vi "add.vi"(0 "reference":refnum<class "Graph.lvclass">, 1 "node":refnum<class "AbstractNode.lvclass">, 2 "point":T1 {"y" format="%.2f"; "x" format="%.2f"}, 5 "error in (no error)":errorcluster) -> (14 "reference out":refnum<class "Graph.lvclass">, 15 "added":bool, 19 "error out":errorcluster)   [LabVIEW 2020, in "Graph.lvclass"]
doc: "public boolean add(Node n, Point2D p)"
uses:
  <resource>/Framework/Providers/Open_GDS/UML/Graph_class/Graph.lvclass
  <resource>/Framework/Providers/Open_GDS/UML/AbstractNode_class/AbstractNode.lvclass
  <resource>/Framework/Providers/Open_GDS/UML/General/Point/Point Point2D.ctl
  <resource>/Framework/Providers/Open_GDS/UML/RectangularNode_class/RectangularNode.lvclass
  C:/Program Files (x86)/National Instruments/LabVIEW 2020/resource/Framework/Providers/Open_GDS/UML/AbstractNode_class/AbstractNode.lvclass
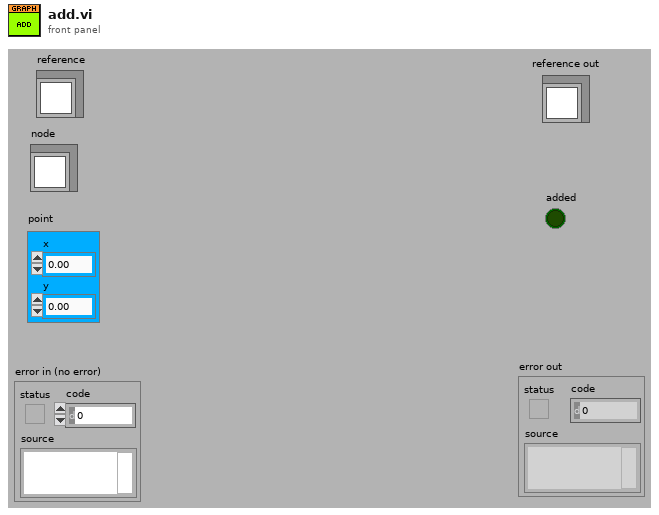
[diagram p1: front panel]
types:
  T1 = typedef "Point Point2D.ctl" = cluster{"x":dbl, "y":dbl}
  T2 = typedef "Graph.lvclass/ObjectAttributes.ctl" = cluster{"nodes":refnum<class "AbstractNode.lvclass">[], "edges":refnum<class "AbstractEdge.lvclass">[], "nodesToBeRemoved":refnum<class "AbstractNode.lvclass">[], "edgesToBeRemoved":refnum<class "AbstractEdge.lvclass">[], "needsLayout":bool, "LayoutNodes":refnum<class "AbstractNode.lvclass">[]}
  T3 = typedef "Rectangle Rectangle2D.ctl" = cluster{"x":dbl, "y":dbl, "width":dbl, "height":dbl}
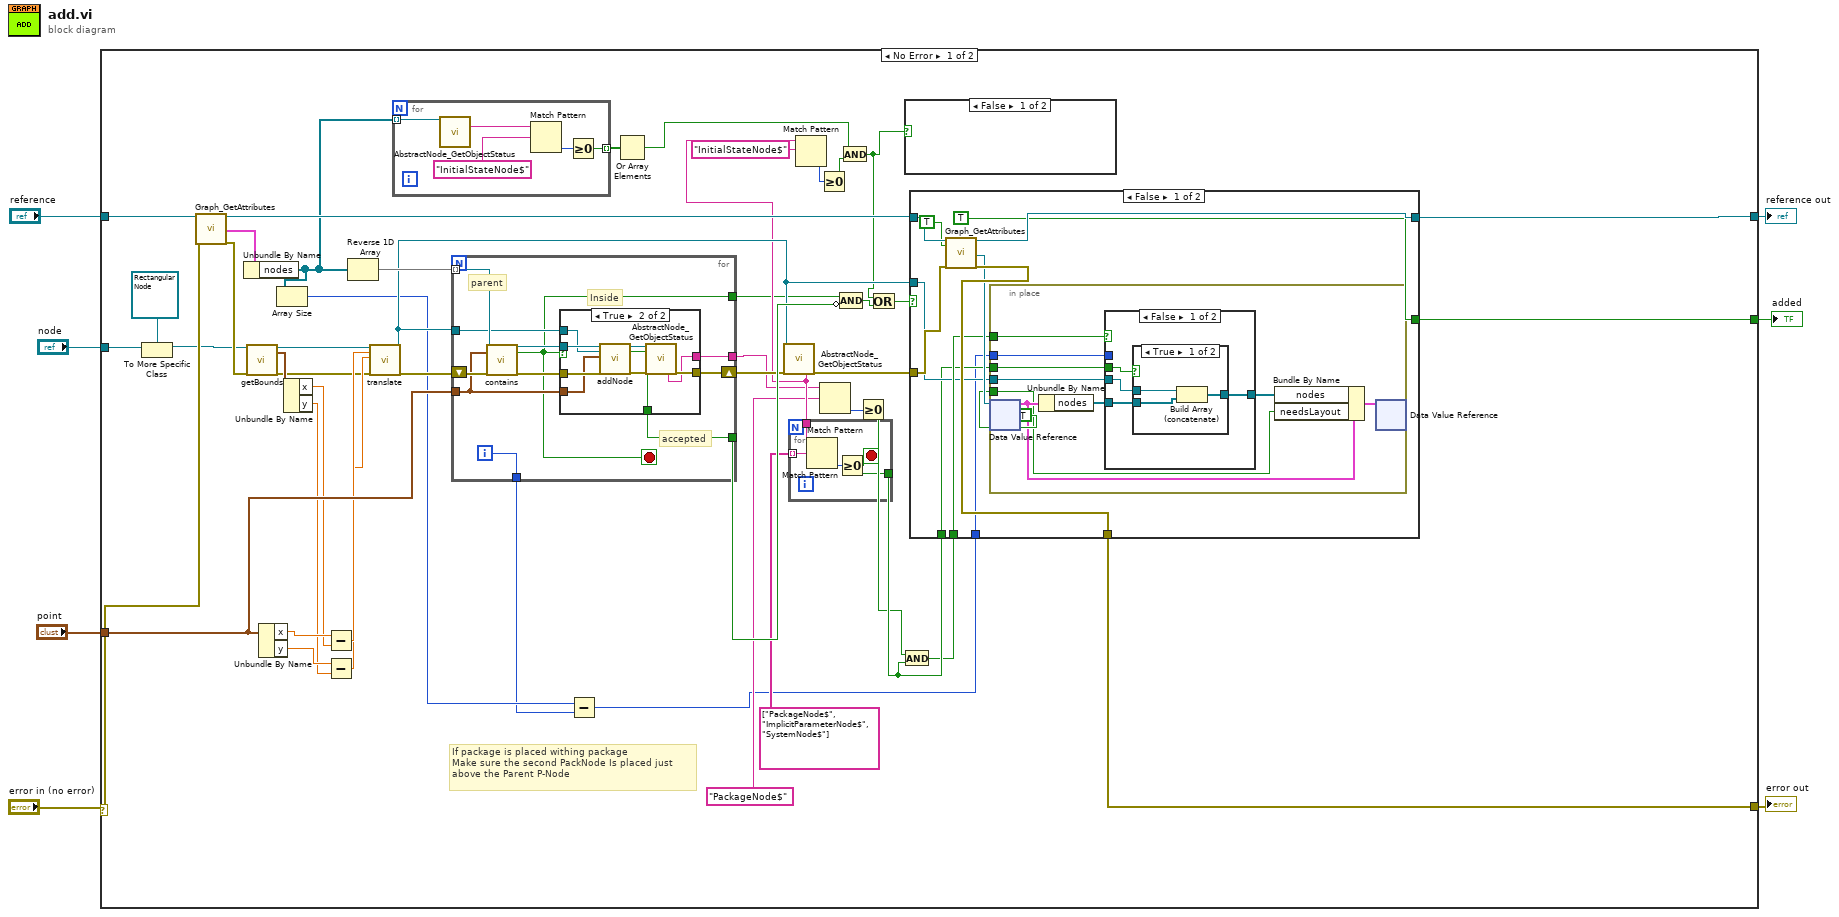
[diagram p0: block diagram]
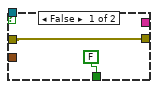
[diagram p2: hidden frame]
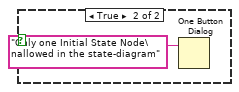
[diagram p3: hidden frame]
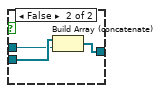
[diagram p4: hidden frame]
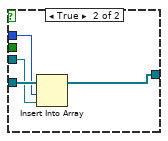
[diagram p5: hidden frame]
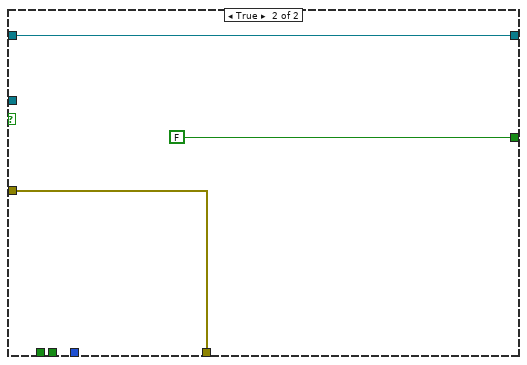
[diagram p6: hidden frame]
diagram:
  n1 = case shown="No Error" "error in (no error)" {
    selector: "error in (no error)" -> [w52 w126]
    tunnel: "reference" -> [w55 w127]
    tunnel: [w54 w126] -> w6
    tunnel: [w53 w127] -> w5
    tunnel: "node" -> [w21 _]
    tunnel: "point" -> [w51 _]
    tunnel: [w50 _] -> w1
    frame No Error {
      # "If package is placed withing package\nMake sure the second PackNode Is placed just\nabove the Parent P-Node"
      n2 = To More Specific Class(target class=refnum<class "RectangularNode.lvclass"> refnum ("reference"), reference=w21) -> (specific class reference=w19:refnum<class "RectangularNode.lvclass">)  [unwired: 1 in, 1 out]
      n3 = call <resource>:"Graph_GetAttributes.vi"("reference in"=w55, "error in (no error)"=w52) -> ("reference out"=w39:refnum<class "Graph.lvclass">, "Data"=w8:T2, "error out"=w36:errorcluster)  [unwired: 1 in, 14 out]
      n4 = Unbundle By Name(w8) -> ("nodes"=w30:refnum<class "AbstractNode.lvclass">[])
      n5 = call-dynamic "getBounds.vi"("reference"=w19, "error in (no error)"=w36) -> ("reference out"=w49:refnum<class "RectangularNode.lvclass">, "bounds"=w47:T3, "error out"=w41:errorcluster)  [unwired: 15 in]
      n6 = Unbundle By Name(w51) -> ("x"=w48:dbl, "y"=w44:dbl)
      n7 = Array Size(array=w30) -> (size(s)=w14:i32)
      n8 = Unbundle By Name(w47) -> ("x"=w46:dbl, "y"=w43:dbl)
      n9 = Subtract(x=w48, y=w46) -> (x-y=w45:dbl)
      n10 = Subtract(x=w44, y=w43) -> (x-y=w42:dbl)
      n11 = Reverse 1D Array(array=w30) -> (reversed array=w35:refnum<class "AbstractNode.lvclass">[])
      n12 = call-dynamic "translate.vi"("reference"=w49, "dx"=w45, "dy"=w42, "error in (no error)"=w41) -> ("reference out"=w32:refnum<class "RectangularNode.lvclass">, "error out"=w40:errorcluster)  [unwired: 14 in]
      n13 = for {
        tunnel: w30 -> [w83] mode=indexing
        tunnel: [w80] -> w27 mode=indexing
        n14 = call <resource>:"AbstractNode_GetObjectStatus.vi"("reference in"=w83) -> ("Class name"=w79:string)  [unwired: 1 in, 17 out]
        n15 = Match Pattern(string=w79, regular expression="InitialStateNode$" ("y")) -> (offset past match=w81:i32)  [unwired: 4 out]
        n16 = Greater Or Equal To 0?(x=w81) -> (x >= 0?=w80:bool)
      }
      n17 = for {
        shift-right: [w60] -> w34
        shift-left: w40 -> [w66]
        tunnel: w35 -> [w65] mode=indexing
        tunnel: [w56] -> w18
        tunnel: w32 -> [w62]
        tunnel: w51 -> [w61]
        tunnel: [w58] -> w38
        tunnel: [w59] -> w17
        tunnel: [w57] -> w13
        i -> [w57]
        stop <- w56 stop-if-true
        # "parent"
        # "accepted"
        # "Inside"
        n18 = call-dynamic "contains.vi"("reference"=w65, "point2D"=w61, "error in (no error)"=w66) -> ("reference out"=w63:refnum<class "AbstractNode.lvclass">, "contains"=w56:bool, "error out"=w64:errorcluster)  [unwired: 14 in]
        n19 = case shown="True" w56 {
          tunnel: w64 -> [w68 w77]
          tunnel: w63 -> [_ w76]
          tunnel: w62 -> [_ w75]
          tunnel: w61 -> [_ w74]
          tunnel: [w68 w71] -> w60
          tunnel: [FALSE ("added") w73] -> w58
          tunnel: [_ w69] -> w59
          frame False {
          }
          frame True {
            n20 = call-dynamic "addNode.vi"("reference"=w76, "node"=w75, "point2D"=w74, "error in (no error)"=w77) -> ("reference out"=w70:refnum<class "AbstractNode.lvclass">, "added"=w73:bool, "error out"=w72:errorcluster)  [unwired: 13 in]
            n21 = call <resource>:"AbstractNode_GetObjectStatus.vi"("reference in"=w70, "error in (no error)"=w72) -> ("Class name"=w69:string, "error out"=w71:errorcluster)  [unwired: 16 out]
          }
        }
      }
      n22 = Subtract(x=w14, y=w13) -> (x-y=w12:i32)
      n23 = Or Array Elements(Boolean array=w27) -> (logical OR=w24:bool)
      n24 = call <resource>:"AbstractNode_GetObjectStatus.vi"("reference in"=w32, "error in (no error)"=w34) -> ("Class name"=w29:string, "error out"=w33:errorcluster)  [unwired: 16 out]
      n25 = for {
        tunnel: [w84] -> w11
        tunnel: w29 -> [w86]
        tunnel: string[] ["PackageNode$", "ImplicitParameterNode$", "SystemNode$"] -> [w85] mode=indexing
        stop <- w84 stop-if-true
        n26 = Match Pattern(string=w86, regular expression=w85) -> (offset past match=w87:i32)  [unwired: 4 out]
        n27 = Greater Or Equal To 0?(x=w87) -> (x >= 0?=w84:bool)
      }
      n28 = Match Pattern(string=w29, regular expression="InitialStateNode$" ("y")) -> (offset past match=w26:i32)  [unwired: 4 out]
      n29 = Greater Or Equal To 0?(x=w26) -> (x >= 0?=w25:bool)
      n30 = Match Pattern(string=w17, regular expression="PackageNode$" ("y")) -> (offset past match=w15:i32)  [unwired: 4 out]
      n31 = And(x=w24, y=w25) -> (x .and. y?=w22:bool)
      n32 = Compound Arithmetic op=AND(w18, invert w38) -> (w37:bool)
      n33 = Greater Or Equal To 0?(x=w15) -> (x >= 0?=w10:bool)
      n34 = Or(x=w22, y=w37) -> (x .or. y?=w23:bool)
      n35 = And(x=w10, y=w11) -> (x .and. y?=w9:bool)
      n36 = case shown="False" w22 {
        frame False {
        }
        frame True {
          n37 = One Button Dialog(message="Only one Initial State Node\nallowed in the state-diagram") -> ()  [unwired: 2 out]
        }
      }
      n38 = case shown="False" w23 {
        tunnel: w39 -> [w99 w125]
        tunnel: [w98 w125] -> w53
        tunnel: [TRUE ("needsLayout") FALSE] -> w50
        tunnel: w33 -> [w95 w123]
        tunnel: [w96 w123] -> w54
        tunnel: w32 -> [w90 _]
        tunnel: w11 -> [w89 _]
        tunnel: w12 -> [w88 _]
        tunnel: w9 -> [w91 _]
        frame False {
          n39 = call <resource>:"Graph_GetAttributes.vi"("reference in"=w99, "OnlyGetDvrReference(False)"=TRUE, "error in (no error)"=w95) -> ("reference out"=w98:refnum<class "Graph.lvclass">, "DataRef"=w93:refnum<data-value>, "error out"=w96:errorcluster)  [unwired: 13 in, 1 out]
          n40 = in-place {
            in-place-border: TRUE ("needsLayout") -> [w105]
            in-place-border: w91 -> [w103]
            in-place-border: w90 -> [w102]
            in-place-border: w89 -> [w101]
            in-place-border: w88 -> [w100]
            n41 = in-place-dvr #1(w93) -> (w108:T2)  [unwired: 1 out]
            n42 = Unbundle By Name(w108) -> ("nodes"=w107:refnum<class "AbstractNode.lvclass">[])
            n43 = case shown="False" w103 {
              tunnel: w107 -> [w112 w122]
              tunnel: [w111 w121] -> w106
              tunnel: w102 -> [w110 w120]
              tunnel: w101 -> [w109 _]
              tunnel: w100 -> [_ w119]
              frame False {
                n44 = case shown="True" w109 {
                  tunnel: w112 -> [w113 w118]
                  tunnel: [w115 w117] -> w111
                  tunnel: w110 -> [w114 w116]
                  frame True {
                    n45 = Build Array (concatenate)(w114, w113) -> (w115:refnum<class "AbstractNode.lvclass">[])
                  }
                  frame False {
                    n46 = Build Array (concatenate)(w118, w116) -> (w117:refnum<class "AbstractNode.lvclass">[])
                  }
                }
              }
              frame True {
                n47 = Insert Into Array(array=w122, index=w119, new element=w120) -> (w121:refnum<class "AbstractNode.lvclass">[])
              }
            }
            n48 = Bundle By Name(cluster=w108, "nodes"=w106, "needsLayout"=w105) -> (w104:T2)
            n49 = in-place-dvr #1(w104) -> ()  [unwired: 2 out]
          }
        }
        frame True {
        }
      }
    }
    frame Error {
    }
  }
  "reference out" <- w5
  "error out" <- w6
  "added" <- w1
